vi "Disconnect.vi"(8 "error in (no error)":errorcluster, 11 "MPLab in":refnum<class "MPLab.lvclass">) -> (0 "error out":errorcluster, 3 "MPLab out":refnum<class "MPLab.lvclass">)   [LabVIEW 2018, in "MPLab.lvlib" / "MPLab.lvclass"]
uses:
  MPLab.lvclass
  builds/Flash Utility.lvlibp/Flash Utility.lvclass
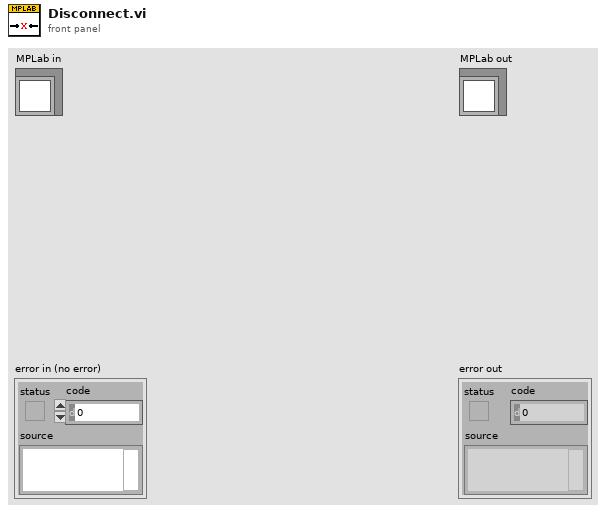
[diagram p1: front panel]
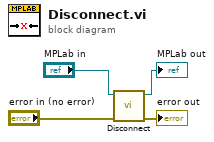
[diagram p0: block diagram]
diagram:
  n1 = call-parent "Disconnect.vi"("error in (no error)"="error in (no error)", "Flash Utility in"="MPLab in") -> ("error out"=→"error out":errorcluster, "Flash Utility out"=→"MPLab out":refnum<class "MPLab.lvclass">)  [unwired: 8 in]
